vi "StreamWaveform.vi"() -> ()   [LabVIEW 2019]
panel:
  in  "First Call":bool
  out "error out":errorcluster
  in  "error in (no error)":errorcluster
  in  "Waveforms":waveform(dbl)[](array[waveform])
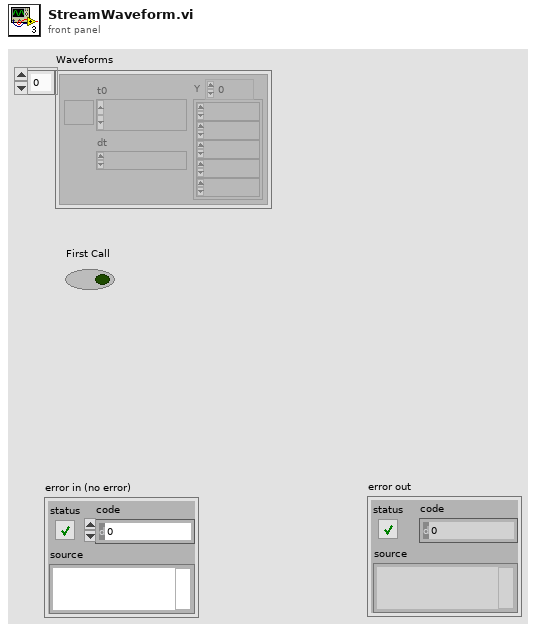
[diagram p1: front panel]
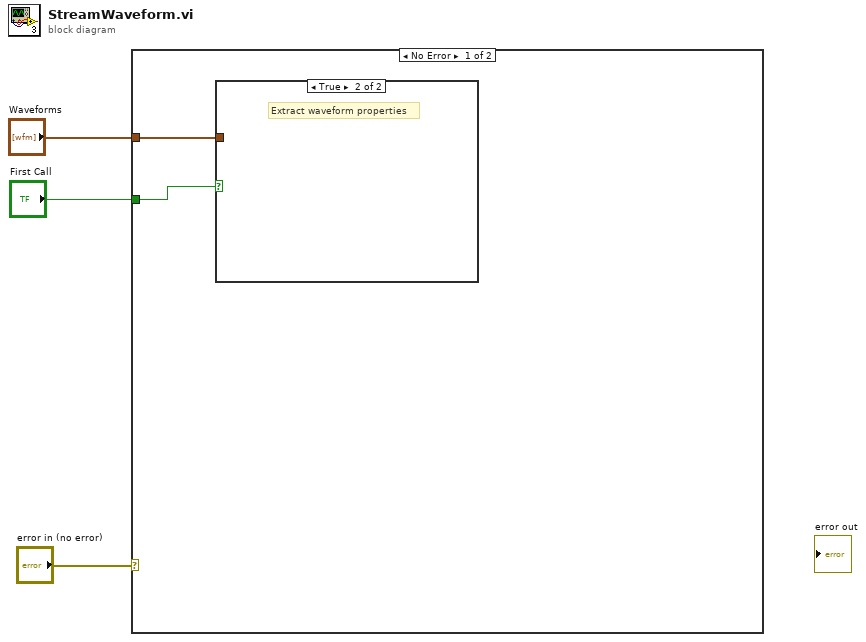
[diagram p0: block diagram]
diagram:
  n1 = case shown="No Error" "error in (no error)" {
    tunnel: "Waveforms" -> [w4 _]
    tunnel: "First Call" -> [w5 _]
    frame No Error {
      n2 = case shown="True" w5 {
        tunnel: w4 -> [_ _]
        frame False {
        }
        frame True {
          # "Extract waveform properties"
        }
      }
    }
    frame Error {
    }
  }
